vi "TestVI1.vi"() -> ()   [LabVIEW 2016, in "test_Setup.lvlib"]
uses:
  test_Setup.lvlib
panel:
  in  "test-ctl":dbl
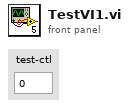
[diagram p1: front panel]
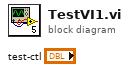
[diagram p0: block diagram]
diagram:
